vi "QTab DEMO.vi"() -> ()   [LabVIEW 2020]
uses:
  QTab Class/QTab Class.lvclass/QTab Class.ctl
  QTab Class/Pag Attribute.ctl
  QTab Class/Read Notifier User Event.vi
  QTab Class/QTab Class.lvclass
panel:
  in  "Set Attribute":bool
  in  "Merage":bool
  in  "Close All":bool
  in  "Sub 3":bool
  in  "Sub 2":bool
  in  "Sub 1":bool
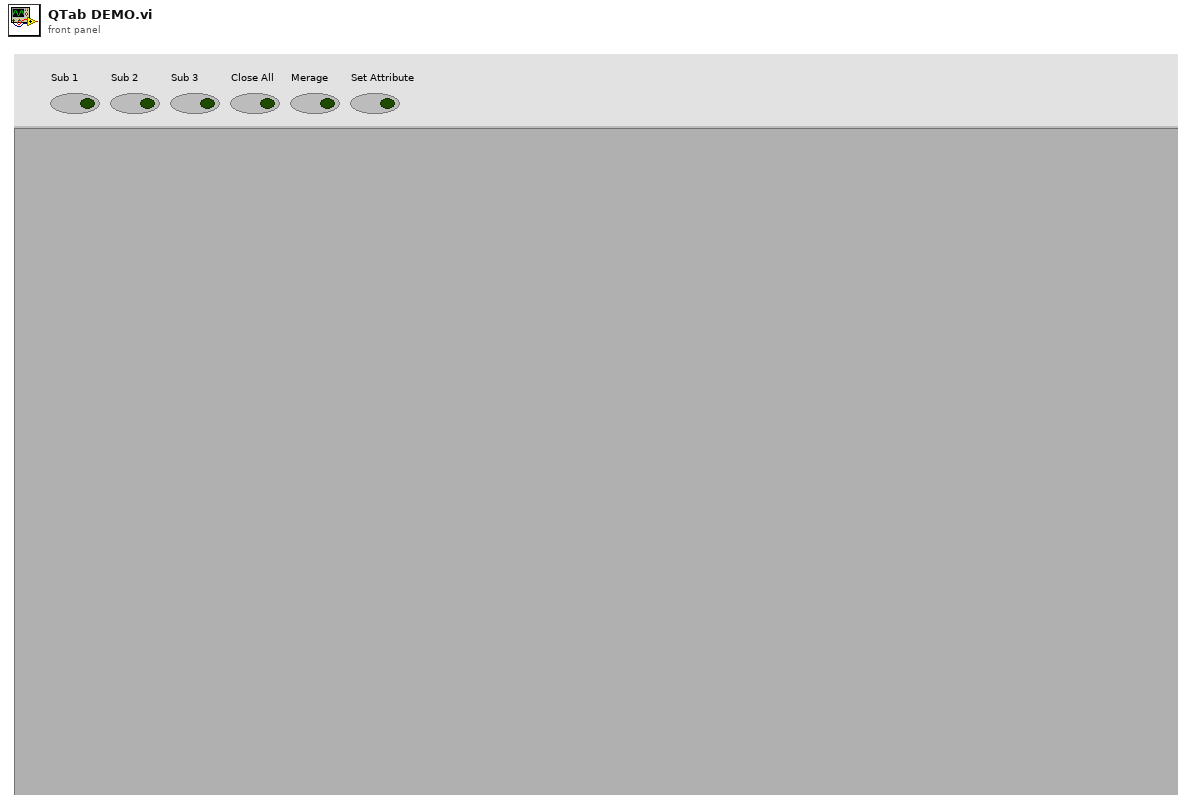
[diagram p1: front panel]
types:
  T1 = typedef "QTab.lvlib/QTab Class.lvclass/Notifier User Event.ctl" = cluster{"Close User Event":refnum<user-event>}
  T2 = typedef "QTab.lvlib/QTab Class.lvclass/Pag Attribute.ctl" = cluster{"VI Refnum":refnum<vi>, "Page Name":string, "Closeable":bool, "Draggable":bool, "Pop-Out":bool}
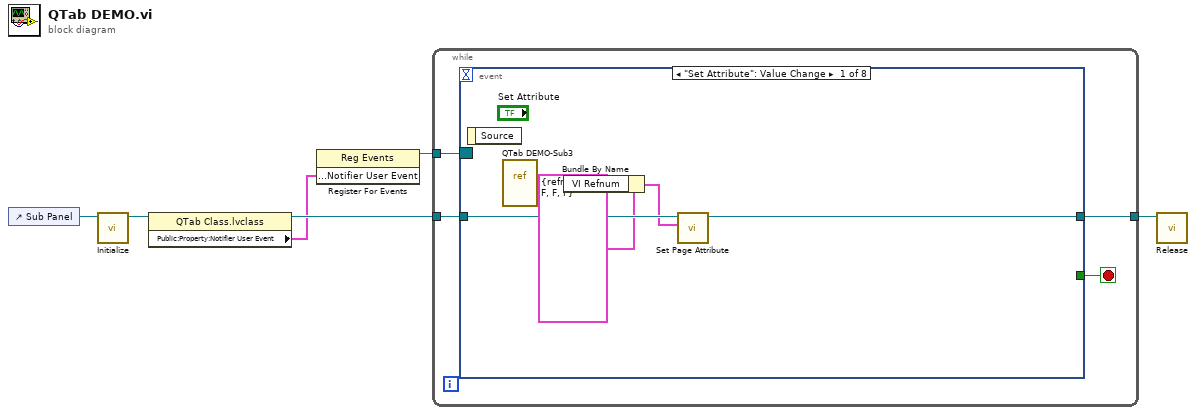
[diagram p0: block diagram]
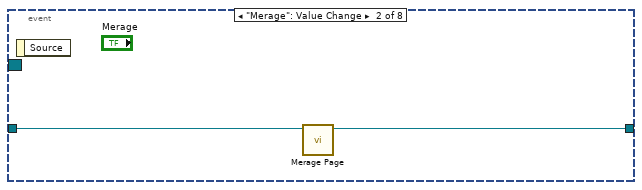
[diagram p2: hidden frame]
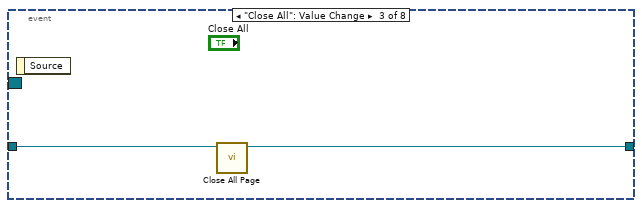
[diagram p3: hidden frame]
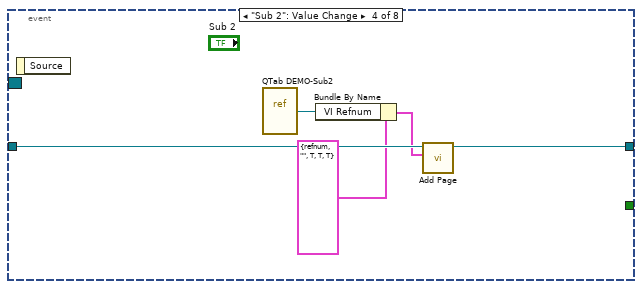
[diagram p4: hidden frame]
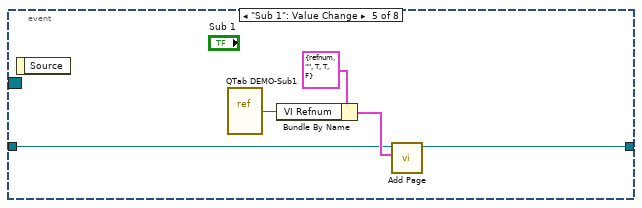
[diagram p5: hidden frame]
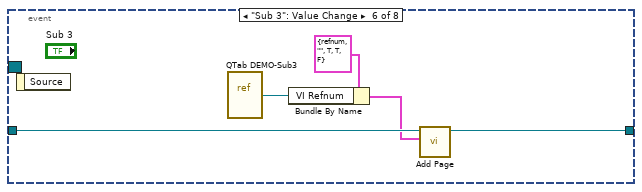
[diagram p6: hidden frame]
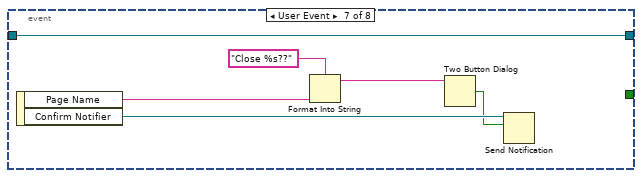
[diagram p7: hidden frame]
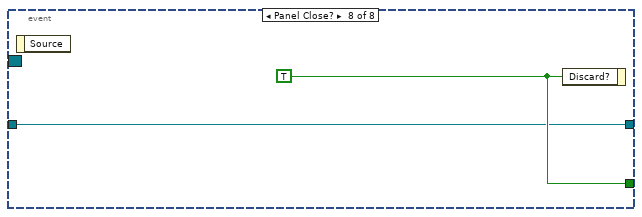
[diagram p8: hidden frame]
diagram:
  n1 = control-ref of="Sub Panel"() -> (w3:refnum<vi>)
  n2 = call "Initialize.vi"("SubPnl Refnum"=w3) -> ("QTab Class out"=w2:refnum<class "QTab Class.lvclass">)  [unwired: 9 in, 1 out]
  n3 = property class="QTab Class.lvclass"(reference=w2) -> (reference out=w6:refnum<class "QTab Class.lvclass">, "Public:Property:Notifier User Event"=w5:T1)  [unwired: 1 in, 1 out]
  n4 = register-events(w5) -> (reference out=w4:refnum<event-registration>)  [unwired: 2 in, 1 out]
  n5 = while {
    tunnel: [w10] -> w1
    tunnel: w6 -> [w8]
    tunnel: w4 -> [w7]
    stop <- w9 stop-if-true
    n6 = event shown="[0] \"Set Attribute\": Value Change" {
      selector: w7 -> [_ _ _ _ _ _ _ _]
      dyn-events: _ -> [_ _ _ _ _ _ _ _]
      timeout: _ -> [_ _ _ _ _ _ _ _]
      tunnel: [w14 w16 w18 w24 w26 w34 w40 w41] -> w10
      tunnel: [_ _ _ _ _ _ _ w42] -> w9
      tunnel: w8 -> [w15 w17 w19 w23 w27 w33 w40 w41]
      event "Set Attribute": Value Change {
        n7 = event-data() -> ()  [unwired: 1 in, 1 out]
        n8 = vi-ref "QTab DEMO-Sub3.vi"() -> (w12:refnum<vi>)
        n9 = Bundle By Name(cluster=T2 {"VI Refnum"=refnum, "Page Name"="", "Closeable"=FALSE, "Draggable"=FALSE, "Pop-Out"=FALSE} ("Pag Attribute"), "VI Refnum"=w12) -> (w11:T2)
        n10 = call "Set Page Attribute.vi"("Pag Attribute"=w11, "QTab Class in"=w15) -> ("QTab Class out"=w14:refnum<class "QTab Class.lvclass">)  [unwired: 8 in, 1 out]
      }
      event "Merage": Value Change {
        n11 = event-data() -> ()  [unwired: 1 in, 1 out]
        n12 = call "Merage Page.vi"("QTab Class in"=w17) -> ("QTab Class out"=w16:refnum<class "QTab Class.lvclass">)  [unwired: 9 in, 1 out]
      }
      event "Close All": Value Change {
        n13 = event-data() -> ()  [unwired: 1 in, 1 out]
        n14 = call "Close All Page.vi"("QTab Class in"=w19) -> ("QTab Class out"=w18:refnum<class "QTab Class.lvclass">)  [unwired: 8 in, 2 out]
      }
      event "Sub 2": Value Change {
        n15 = event-data() -> ()  [unwired: 1 in, 1 out]
        n16 = vi-ref "QTab DEMO-Sub2.vi"() -> (w21:refnum<vi>)
        n17 = Bundle By Name(cluster=T2 {"VI Refnum"=refnum, "Page Name"="", "Closeable"=TRUE, "Draggable"=TRUE, "Pop-Out"=TRUE} ("Pag Attribute"), "VI Refnum"=w21) -> (w20:T2)
        n18 = call "Add Page.vi"("Pag Attribute"=w20, "QTab Class in"=w23) -> ("QTab Class out"=w24:refnum<class "QTab Class.lvclass">)  [unwired: 8 in, 1 out]
      }
      event "Sub 1": Value Change {
        n19 = event-data() -> ()  [unwired: 1 in, 1 out]
        n20 = vi-ref "QTab DEMO-Sub1.vi"() -> (w25:refnum<vi>)
        n21 = Bundle By Name(cluster=T2 {"VI Refnum"=refnum, "Page Name"="", "Closeable"=TRUE, "Draggable"=TRUE, "Pop-Out"=FALSE} ("Pag Attribute"), "VI Refnum"=w25) -> (w29:T2)
        n22 = call "Add Page.vi"("Pag Attribute"=w29, "QTab Class in"=w27) -> ("QTab Class out"=w26:refnum<class "QTab Class.lvclass">)  [unwired: 8 in, 1 out]
      }
      event "Sub 3": Value Change {
        n23 = event-data() -> ()  [unwired: 1 in, 1 out]
        n24 = vi-ref "QTab DEMO-Sub3.vi"() -> (w31:refnum<vi>)
        n25 = Bundle By Name(cluster=T2 {"VI Refnum"=refnum, "Page Name"="", "Closeable"=TRUE, "Draggable"=TRUE, "Pop-Out"=FALSE} ("Pag Attribute"), "VI Refnum"=w31) -> (w30:T2)
        n26 = call "Add Page.vi"("Pag Attribute"=w30, "QTab Class in"=w33) -> ("QTab Class out"=w34:refnum<class "QTab Class.lvclass">)  [unwired: 8 in, 1 out]
      }
      event User Event {
        n27 = event-data() -> ("Page Name"=w39:string, "Confirm Notifier"=w36:refnum<notifier>)  [unwired: 1 in]
        n28 = Format Into String(format string="Close %s??", w39) -> (resulting string=w37:string)  [unwired: 2 in, 1 out]
        n29 = Two Button Dialog(message=w37) -> (T button?=w35:bool)  [unwired: 2 in]
        n30 = Send Notification(notification=w35, notifier=w36) -> ()  [unwired: 1 in, 2 out]
      }
      event Panel Close? {
        w42 = TRUE ("Discard?")
        n31 = event-data() -> ()  [unwired: 1 in, 1 out]
        n32 = event-data("Discard?"=w42) -> ()  [unwired: 1 in, 1 out]
      }
    }
  }
  n33 = call "Release.vi"("QTab Class in"=w1) -> ()  [unwired: 10 in, 1 out]
